vi "Shooter Check.vi"(8 "MaxSonar Distance to Castle":dbl, 9 "IR Distance to Castle":dbl, 11 "Straight/tilt?":dbl) -> (3 "Boolean":bool=TRUE)   [LabVIEW 2015]
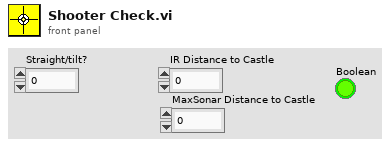
[diagram p1: front panel]
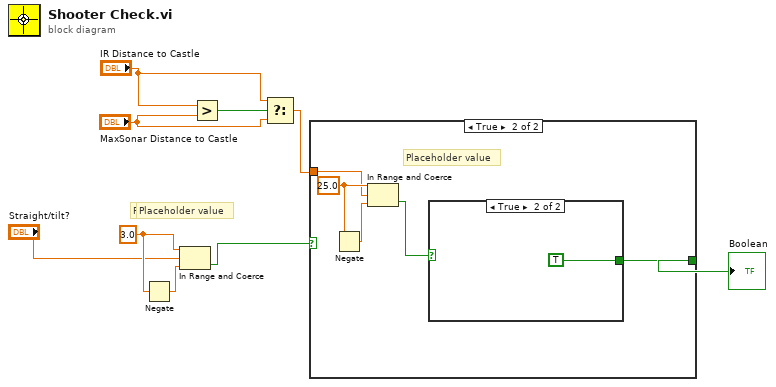
[diagram p0: block diagram]
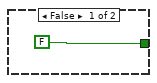
[diagram p2: hidden frame]
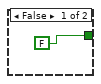
[diagram p3: hidden frame]
diagram:
  w2 = 3.0 ("upper limit")
  # "Placeholder value"
  # "Placeholder value"
  n1 = Negate(x=w2) -> (-x=w9:dbl)
  n2 = In Range and Coerce(upper limit=w2, x="Straight/tilt?", lower limit=w9) -> (In Range?=w8:bool)  [unwired: 1 out]
  n3 = Greater?(x="IR Distance to Castle", y="MaxSonar Distance to Castle") -> (0:w6:bool)
  n4 = Select(t="IR Distance to Castle", s=w6, f="MaxSonar Distance to Castle") -> (s? t:f=w3:dbl)
  n5 = case shown="True" w8 {
    tunnel: [FALSE w12] -> w7
    tunnel: w3 -> [_ w11]
    frame False {
    }
    frame True {
      w15 = 25.0 ("upper limit")
      # "Placeholder value"
      n6 = Negate(x=w15) -> (-x=w14:dbl)
      n7 = In Range and Coerce(upper limit=w15, x=w11, lower limit=w14) -> (In Range?=w13:bool)  [unwired: 1 out]
      n8 = case shown="True" w13 {
        tunnel: [FALSE TRUE] -> w12
        frame False {
        }
        frame True {
        }
      }
    }
  }
  "Boolean" <- w7
